vi "Write min record length (100 samples).vi"(8 "error in (no error)":errorcluster, 10 "min record length (100 samples)":i32=100, 11 "Configure Acquisition Record Msg in":refnum<class "Configure Acquisition Record Msg.lvclass">) -> (0 "error out":errorcluster, 3 "Configure Acquisition Record Msg out":refnum<class "Configure Acquisition Record Msg.lvclass">)   [LabVIEW 2015, in "CS++Scope.lvlib" / "Configure Acquisition Record Msg.lvclass"]
uses:
  Configure Acquisition Record Msg.lvclass
  Configure Acquisition Record Msg.lvclass/Configure Acquisition Record Msg.ctl
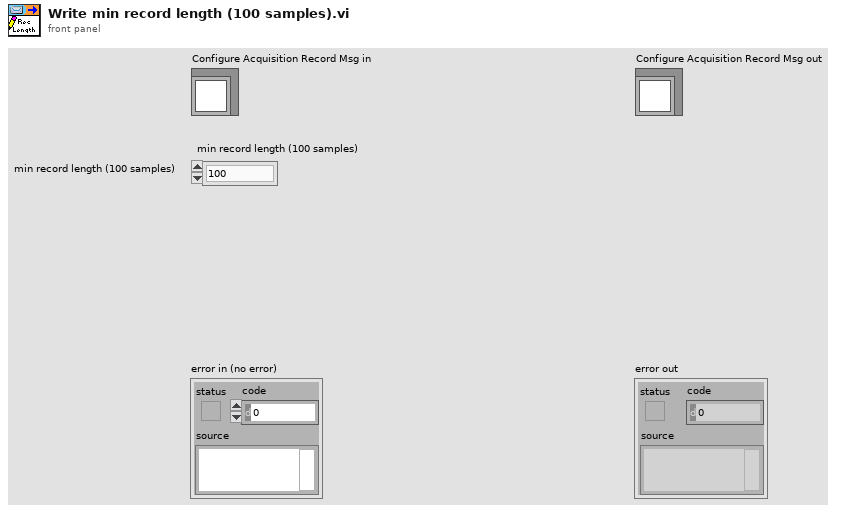
[diagram p1: front panel]
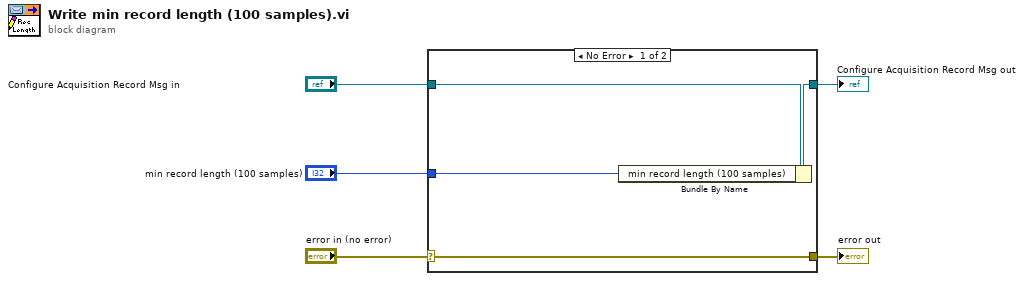
[diagram p0: block diagram]
diagram:
  n1 = case shown="No Error" "error in (no error)" {
    selector: "error in (no error)" -> [w9 w10]
    tunnel: [w9 w10] -> w4
    tunnel: [w7 w11] -> w2
    tunnel: "Configure Acquisition Record Msg in" -> [w8 w11]
    tunnel: "min record length (100 samples)" -> [w6 _]
    frame No Error {
      n2 = Bundle By Name(cluster=w8, "min record length (100 samples)"=w6) -> (w7:refnum<class "Configure Acquisition Record Msg.lvclass">)
    }
    frame Error {
    }
  }
  "error out" <- w4
  "Configure Acquisition Record Msg out" <- w2
